vi "LINX - I2C Write Benchmark.vi"() -> ()   [LabVIEW 2019]
uses:
  <vilib>/MakerHub/LINX/Private/Local IO/LinxI2cWrite.vi
  <vilib>/MakerHub/LINX/Public/Utilities/Check Channel.vi
  <vilib>/MakerHub/LINX/Public/Utilities/Open Local.vi
  <vilib>/MakerHub/LINX/Private/Utilties/Generate Error.vi
  <vilib>/MakerHub/LINX/LMH-LINX.lvlib
panel:
  in  "Warmup Iterations":i32=100
  out "Chart":dbl(graph)
  in  "Stop Button":bool
  in  "Benchmark Iterations":i32=1000
  out "Samples Per Second":i32
  in  "I2C Channel":u8=2
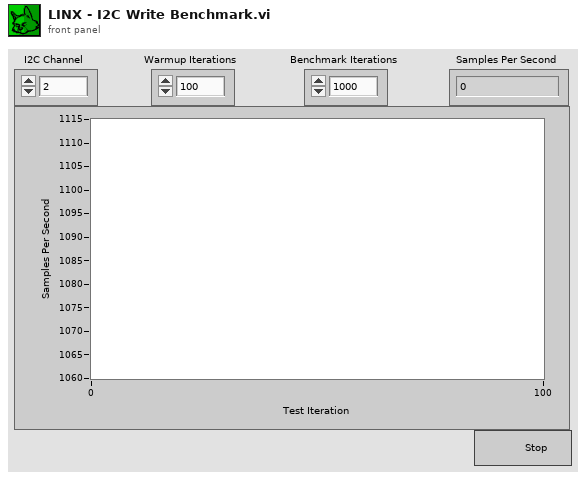
[diagram p1: front panel]
types:
  T1 = typedef "LMH-LINX.lvlib/LINX Ref.ctl" = cluster{"IO":T2, "Interface":T3, "LINX Device Config":T4}
  T2 = typedef "LMH-LINX.lvlib/Platform.ctl" = enum16{"Remote", "Local"}
  T3 = typedef "LMH-LINX.lvlib/Interface.ctl" = enum16{"Serial", "TCP"}
  T4 = typedef "LMH-LINX.lvlib/Device.lvlib/LINX Device Config.ctl" = cluster{"Interface":T3, "COM Port":refnum<visa-resource-name>, "TCP Configuration":T5, "Device Family":u8, "Device ID":u8, "Device Name":string, "TCP Ref":refnum<k5>, "Channels":T6}
  T5 = typedef "LMH-LINX.lvlib/Device.lvlib/TCP Config.ctl" = cluster{"IP Address":string, "Port":u16}
  T6 = typedef "LMH-LINX.lvlib/Channels.ctl" = cluster{"DI":u8[], "DO":u8[], "AI":u8[], "AO":u8[], "PWM":u8[], "QE":u8[], "UART":u8[], "I2C 2":u8[], "SPI":u8[], "CAN":u8[], "Servo":u8[], "AI Ref (V)":dbl, "AI Resolution (Bits)":u8, "AO Ref (V)":dbl, "AO Resolution (Bits)":u8}
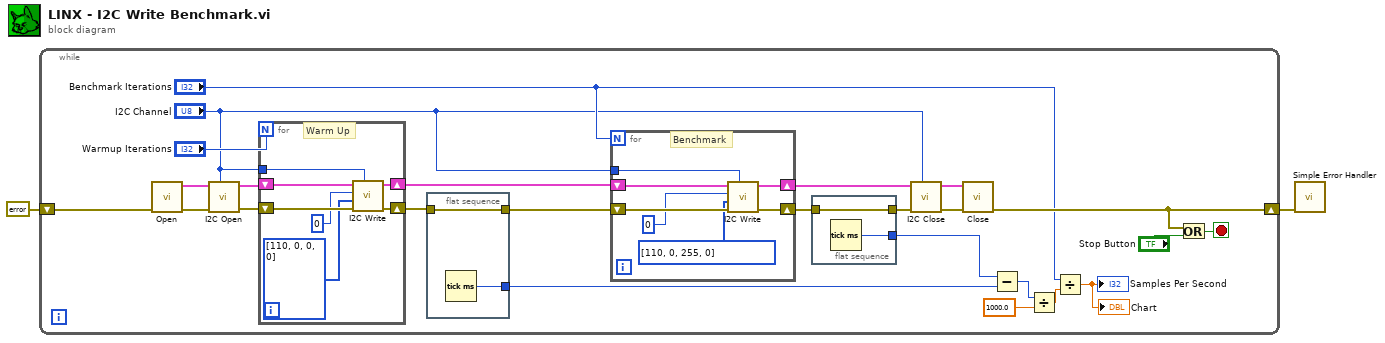
[diagram p0: block diagram]
diagram:
  n1 = while {
    shift-right: [w23] -> w2
    shift-left: errorcluster {"status"=FALSE, "code"=0, "source"=""} ("Error Out") -> [w21]
    stop <- w13 stop-if-true
    n2 = call-poly <vilib>:"Open.vi"("Error In"=w21) -> ("Error Out"=w11:errorcluster, "LINX Resource"=w12:T1)  [unwired: 8 in, 1 out]
    n3 = call <vilib>:"I2C Open.vi"("I2C Channel (0)"="I2C Channel", "Error In"=w11, "LINX Resource"=w12) -> ("Error Out"=w10:errorcluster, "LINX Resource"=w9:T1)  [unwired: 7 in]
    n4 = for {
      N: "Warmup Iterations" -> [_]
      shift-right: [w34] -> w25
      shift-left: w9 -> [w33]
      shift-right: [w32] -> w26
      shift-left: w10 -> [w31]
      tunnel: "I2C Channel" -> [w30]
      # "Warm Up"
      n5 = call <vilib>:"I2C Write.vi"("I2C Channel"=w30, "Error In"=w31, "Data"=u8[] [110, 0, 0, 0], "I2C Slave Address (0)"=u8 0, "LINX Resource"=w33) -> ("Error Out"=w32:errorcluster, "LINX Resource"=w34:T1)  [unwired: 5 in]
    }
    n6 = flat-sequence {
      tunnel: [w45] -> w27
      tunnel: w26 -> [w45]
      tunnel: [w44] -> w16
      frame #0 {
        n7 = Tick Count (ms)() -> (millisecond timer value=w44:u32)
      }
    }
    n8 = for {
      N: "Benchmark Iterations" -> [_]
      shift-right: [w38] -> w4
      shift-left: w25 -> [w41]
      shift-right: [w39] -> w8
      shift-left: w27 -> [w40]
      tunnel: "I2C Channel" -> [w37]
      # "Benchmark"
      n9 = call <vilib>:"I2C Write.vi"("I2C Channel"=w37, "Error In"=w40, "Data"=u8[] [110, 0, 255, 0], "I2C Slave Address (0)"=u8 0, "LINX Resource"=w41) -> ("Error Out"=w39:errorcluster, "LINX Resource"=w38:T1)  [unwired: 5 in]
    }
    n10 = flat-sequence {
      tunnel: [w43] -> w7
      tunnel: w8 -> [w43]
      tunnel: [w42] -> w17
      frame #0 {
        n11 = Tick Count (ms)() -> (millisecond timer value=w42:u32)
      }
    }
    n12 = call <vilib>:"I2C Close.vi"("I2C Channel (0)"="I2C Channel", "Error In"=w7, "LINX Resource"=w4) -> ("Error Out"=w6:errorcluster, "LINX Resource"=w5:T1)  [unwired: 7 in]
    n13 = call <vilib>:"Close.vi"("Error In"=w6, "LINX Resource"=w5) -> ("Error Out"=w23:errorcluster)  [unwired: 9 in]
    n14 = Subtract(x=w17, y=w16) -> (x-y=w20:u32)
    n15 = Divide(x=w20, y=1000.0) -> (x/y=w19:dbl)
    n16 = Divide(x="Benchmark Iterations", y=w19) -> (x/y=→"Chart" →"Samples Per Second":dbl)
    n17 = Or(x=w23, y="Stop Button") -> (x .or. y?=w13:bool)
  }
  n18 = call <vilib>:"Simple Error Handler.vi"("error in (no error)"=w2) -> ()  [unwired: 4 in, 5 out]
